vi "Clamp with AET subVI.vi"(6 "Centroid of blob":dbl[][](array[numeric]) format="%.2f", 7 "Angle (Pixel)":dbl, 8 "error in (no error)":errorcluster, 9 "Clamp param":T1, 10 "All straight Edges":cluster{"Edge Information":T2[]}[](array[cluster]) {"Edge Information"."Distance (Real-World)" format="%.2f"; "Edge Information"."Location (Real-World)"."Y" format="%.2g"; "Edge Information"."Location (Real-World)"."X" format="%.2f"; "Edge Information"."Noise" format="%.2f"; "Edge Information"."Location (Pixel)"."Y" format="%.2g"; "Edge Information"."Location (Pixel)"."X" format="%.2f"; "Edge Information"."Strength" format="%.2f"; "Edge Information"."Distance (Pixel)" format="%.2f"}, 11 "Gray Level Image":T3) -> (0 "error out":errorcluster, 2 "CG":sgl format="%.2f", 3 "Image Out":T3, 4 "Edge points CG":cluster{"X":sgl, "Y":sgl}[](array[cluster]) {"Y" format="%.2f"; "X" format="%.2f"}, 5 "Edge points Height":cluster{"X":sgl, "Y":sgl}[](array[cluster]))   [LabVIEW 2019, in "Algorithm.lvclass"]
uses:
  FrameworkOverrides/Algorithm.lvclass
  <vilib>/vision/Measure.llb/Edge Polarity.ctl
  <vilib>/vision/Measure.llb/Edge Options.ctl
  <vilib>/vision/NI_Vision_Development_Module.lvlib
  <vilib>/vision/Measure.llb/Edge New.ctl
  <vilib>/vision/Image Controls.llb/IMAQ Image.ctl
panel:
  # "INPUTS"
  # "OUTPUTS"
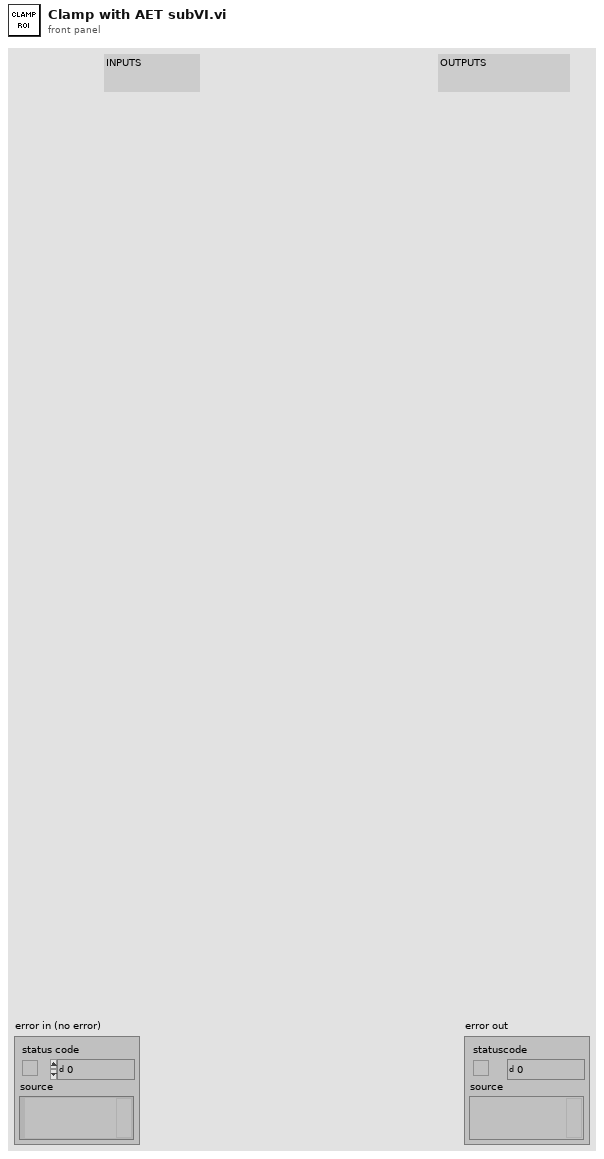
[diagram p1: front panel]
types:
  T1 = cluster{"Start x offset":sgl, "End x offset":sgl, "Start y offset":sgl, "End y offset":sgl, "Carrier offset":sgl, "Height":sgl, "X left":sgl, "X right":sgl, "Angle":sgl}
  T2 = typedef "Edge New.ctl" = cluster{"Location (Pixel)":cluster{"X":sgl, "Y":sgl}, "Location (Real-World)":cluster{"X":sgl, "Y":sgl}, "Distance (Pixel)":dbl, "Distance (Real-World)":dbl, "Strength":dbl, "Noise":dbl, "Rising?":bool}
  T3 = typedef "IMAQ Image.ctl" = refnum<image>
  T4 = cluster{"Point 1":cluster{"X":sgl, "Y":sgl}, "Point 2":cluster{"X":sgl, "Y":sgl}}
  T5 = cluster{"Contrast":i32, "Filter width":i32, "Steepness":i32, "Subsampling Ratio":u32, "Show Search Area":bool, "Show Search Lines":bool, "Show Edges Found":bool, "Show Result":bool}
  T6 = typedef "IMAQ Rectangle" = cluster{"Left":i32, "Top":i32, "Right":i32, "Bottom":i32, "Rotation":dbl}
  T7 = typedef "Edge Options.ctl" = cluster{"Edge Polarity":T8, "Kernel Size":u32, "Width":u32, "Minimum Edge Strength":sgl, "Interpolation Type":enum32{"Zero Order", "Bilinear", "Quadratic", "Cubic", "Bilinear Fixed"}, "Data Processing Method":enum32{"Average", "Median"}}
  T8 = typedef "Edge Polarity.ctl" = u32
  T9 = enum16{"Get First Edge", "Get First + Last Edge", "Get All Edges", "Get Best Edge"}
  T10 = cluster{"Left":i32, "Right":i32, "Top ":i32, "Bottom":i32, "Angle":dbl}
  T11 = typedef "ROI Descriptor" = cluster{"Global Rectangle":i32[], "Contours":cluster{"ID":enum32{"External", "Internal"}, "Type":u32, "Coordinates":i32[]}[]}
  T12 = cluster{"Left":i32, "Top":i32, "Right":i32, "Bottom":i32}
  T13 = cluster{"Location (Pixel)":cluster{"X":sgl, "Y":sgl}, "Point 2":cluster{"X":sgl, "Y":sgl}}
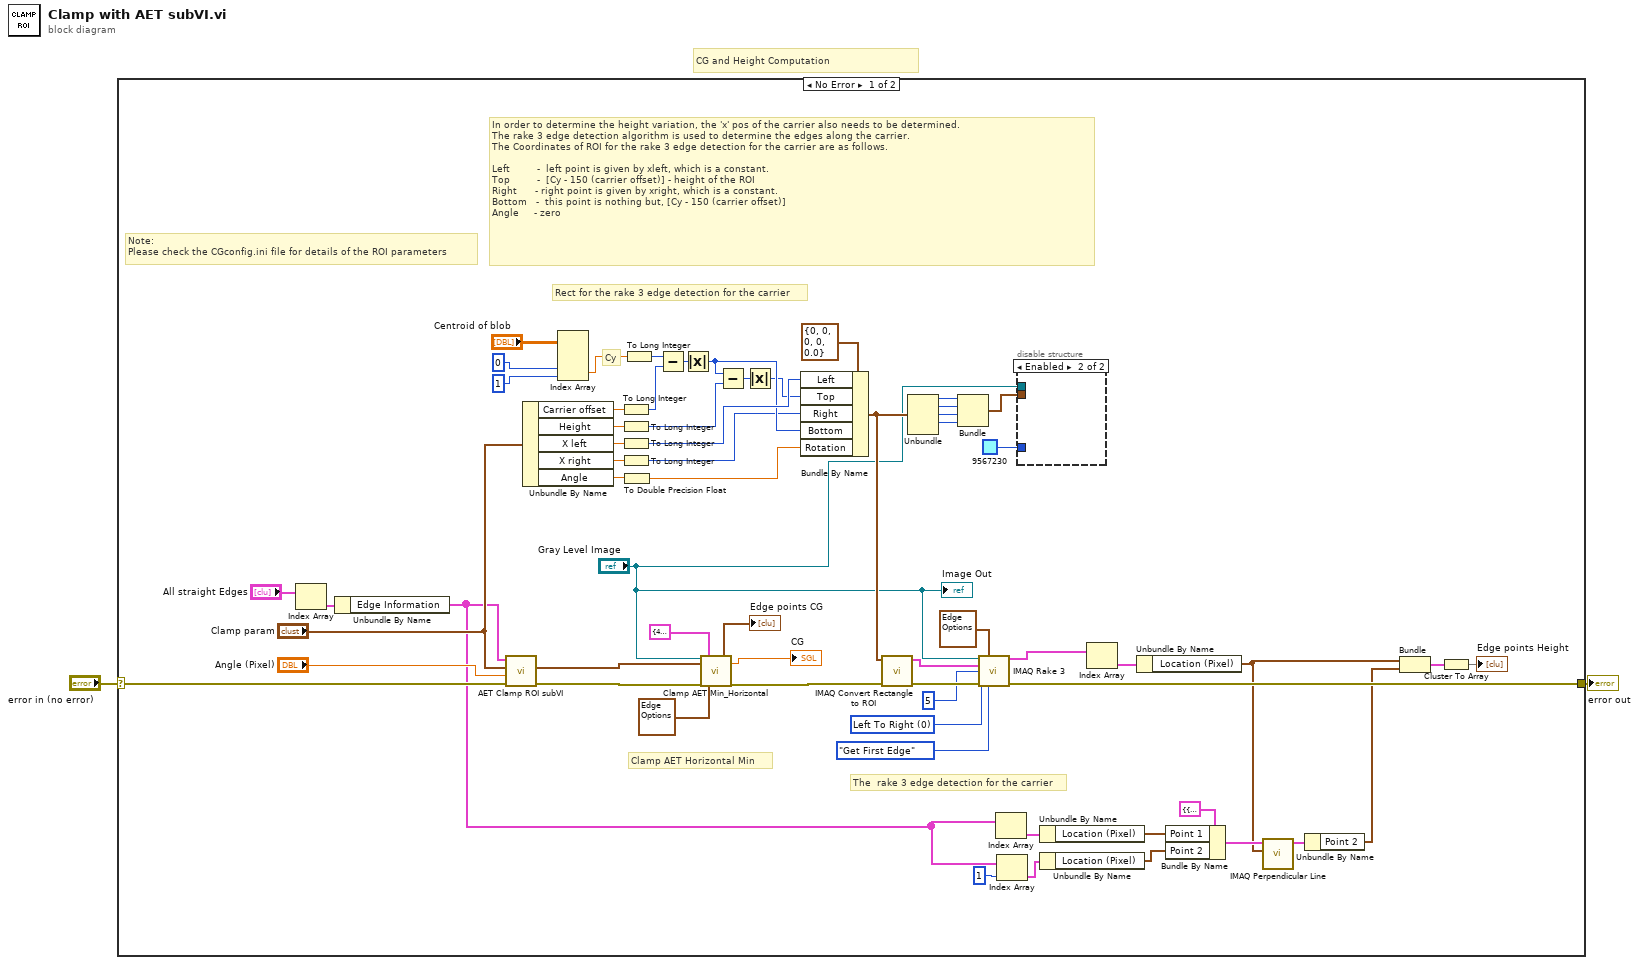
[diagram p0: block diagram]
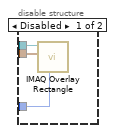
[diagram p2: hidden frame]
diagram:
  # "CG and Height Computation"
  n1 = case shown="No Error" "error in (no error)" {
    selector: "error in (no error)" -> [w55 w68]
    tunnel: [w62 w68] -> w2
    frame No Error {
      w58 = u16 0 items=["Left To Right", "Right To Left", "Top To Bottom", "Bottom To Top"] ("Scan Direction")
      # "Note:\nPlease check the CGconfig.ini file for details of the ROI parameters"
      # "Cy"
      # "In order to determine the height variation, the 'x' pos of the carrier also needs to be determined.\nThe rake 3 edge detection algorithm is used to determine the edges along the carrier.\nThe Coordinates of ROI for the rake 3 edge detection for the carrier are as follows.\n\nLeft         -  left point is given by xleft, which is a constant.\nTop         -  [Cy - 150 (carrier offset)] - height of the ROI \nRight      - right point is given by xright, which is a constant.\nBottom   -  this point is nothing but, [Cy - 150 (carrier offset)]\nAngle     - zero"
      # "Clamp AET Horizontal Min"
      # "Rect for the rake 3 edge detection for the carrier"
      # "The  rake 3 edge detection for the carrier"
      n2 = Index Array(array="All straight Edges") -> (element=w63:cluster{"Edge Information":T2[]})  [unwired: 1 in]
      n3 = Unbundle By Name(w63) -> ("Edge Information"=w13:T2[])
      n4 = call "AET Clamp ROI subVI.vi"("error in (no error)"=w55, "Angle (Pixel)"="Angle (Pixel)", "Clamp param"="Clamp param", "Edge Information"=w13) -> ("error out"=w19:errorcluster, "ROI for AET Clamp"=w24:T10)  [unwired: 5 in, 1 out]
      n5 = Unbundle By Name("Clamp param") -> ("Carrier offset"=w53:sgl, "Height"=w52:sgl, "X left"=w50:sgl, "X right"=w49:sgl, "Angle"=w48:sgl)
      n6 = Index Array(array="Centroid of blob", index (row) #2=0 ("y"), index (col) #2=1 ("y")) -> (element #2=w43:dbl)  [unwired: 2 in, 1 out]
      n7 = To Long Integer(number=w53) -> (32bit integer=w47:i32)
      n8 = To Long Integer(number=w52) -> (32bit integer=w51:i32)
      n9 = To Long Integer(number=w50) -> (32bit integer=w41:i32)
      n10 = To Long Integer(number=w49) -> (32bit integer=w36:i32)
      n11 = To Double Precision Float(number=w48) -> (double precision float=w35:dbl)
      n12 = To Long Integer(number=w43) -> (32bit integer=w46:i32)
      n13 = Subtract(x=w46, y=w47) -> (x-y=w40:i32)
      n14 = Absolute Value(x=w40) -> (abs(x)=w38:i32)
      n15 = call "Clamp AET Min_Horizontal.vi"("Image"="Gray Level Image", "Rectangle"=w24, "error in (no error)"=w19, "Settings"=T5 {"Contrast"=40, "Filter width"=4, "Steepness"=2, "Subsampling Ratio"=5, "Show Search Area"=FALSE, "Show Search Lines"=FALSE, "Show Edges Found"=FALSE, "Show Result"=TRUE}, "Edge Options"=T7 {"Edge Polarity"=0, "Kernel Size"=3, "Width"=3, "Minimum Edge Strength"=50.0, "Interpolation Type"=enum."Bilinear Fixed", "Data Processing Method"=enum."Average"}) -> ("Edge Coordinates"=→"Edge points CG":cluster{"X":sgl, "Y":sgl}[], "Distance"=→"CG":sgl, "error out"=w18:errorcluster)  [unwired: 6 in, 6 out]
      n16 = Subtract(x=w38, y=w51) -> (x-y=w39:i32)
      n17 = Absolute Value(x=w39) -> (abs(x)=w37:i32)
      n18 = Bundle By Name(cluster=T6 {"Left"=0, "Top"=0, "Right"=0, "Bottom"=0, "Rotation"=0.0} ("Rectangle"), "Left"=w41, "Top"=w37, "Right"=w36, "Bottom"=w38, "Rotation"=w35) -> (w32:T6)
      n19 = call "IMAQ Convert Rectangle to ROI"("error in (no error)"=w18, "Rectangle"=w32) -> ("error out"=w60:errorcluster, "ROI Descriptor"=w34:T11)  [unwired: 7 in]
      n20 = Unbundle(w32) -> ("Left"=w31:i32, "Top"=w30:i32, "Right"=w29:i32, "Bottom"=w28:i32)  [unwired: 1 out]
      n21 = Bundle("Left"=w31, "Top"=w30, "Right"=w29, "Bottom"=w28) -> (w27:T12)  [unwired: 1 in]
      n22 = call "IMAQ Rake 3"("Image"="Gray Level Image", "Edge Options"=T7 {"Edge Polarity"=0, "Kernel Size"=3, "Width"=3, "Minimum Edge Strength"=50.0, "Interpolation Type"=enum."Bilinear Fixed", "Data Processing Method"=enum."Average"}, "ROI Descriptor"=w34, "Step Size"=u32 5, "Scan Direction"=w58, "error in (no error)"=w60, "Process"=T9."Get First Edge") -> ("First Edges"=w17:T2[], "error out"=w62:errorcluster)  [unwired: 5 in, 2 out]
      n23 = Index Array(array=w13) -> (element=w15:T2)  [unwired: 1 in]
      n24 = Index Array(array=w13, index=1) -> (element=w14:T2)
      n25 = disable-structure shown="Enabled" {
        disable-tunnel: w27 -> [w67 _]
        disable-tunnel: u32 9567230 ("Color") -> [w66 _]
        disable-tunnel: "Gray Level Image" -> [w65 _]
        frame Disabled {
          n26 = call "IMAQ Overlay Rectangle"("Color"=w66, "Rectangle"=w67, "Image"=w65) -> ()  [unwired: 7 in, 2 out]
        }
        frame Enabled {
        }
      }
      n27 = Unbundle By Name(w15) -> ("Location (Pixel)"=w10:cluster{"X":sgl, "Y":sgl})
      n28 = Unbundle By Name(w14) -> ("Location (Pixel)"=w9:cluster{"X":sgl, "Y":sgl})
      n29 = Index Array(array=w17) -> (element=w16:T2)  [unwired: 1 in]
      n30 = Unbundle By Name(w16) -> ("Location (Pixel)"=w6:cluster{"X":sgl, "Y":sgl})
      n31 = Bundle By Name(cluster=T4 {"Point 1"={"X"=0.0, "Y"=0.0}, "Point 2"={"X"=0.0, "Y"=0.0}} ("Line"), "Point 1"=w10, "Point 2"=w9) -> (w8:T4)
      n32 = call "IMAQ Perpendicular Line"("Point"=w6, "Line"=w8) -> ("Perpendicular Line"=w7:T4)  [unwired: 7 in, 2 out]
      n33 = Unbundle By Name(w7) -> ("Point 2"=w5:cluster{"X":sgl, "Y":sgl})
      n34 = Bundle("Location (Pixel)"=w6, "Point 2"=w5) -> (w4:T13)  [unwired: 1 in]
      n35 = Cluster To Array(cluster=w4) -> (array=→"Edge points Height":cluster{"X":sgl, "Y":sgl}[])
      "Image Out" <- "Gray Level Image"
    }
    frame Error {
    }
  }
  "error out" <- w2
